vi "read single line.vi"(8 "error in (no error)":errorcluster, 11 "USB IO in":refnum<class "USB IO.lvclass">) -> (0 "error out":errorcluster, 2 "data":bool, 3 "USB IO out":refnum<class "USB IO.lvclass">)   [LabVIEW 2025, in "USB IO.lvclass"]
uses:
  USB IO.lvclass
  USB IO.lvclass/USB IO.ctl
  <vilib>/DAQmx/read.llb/DAQmx Read (Digital Bool 1Line 1Point).vi
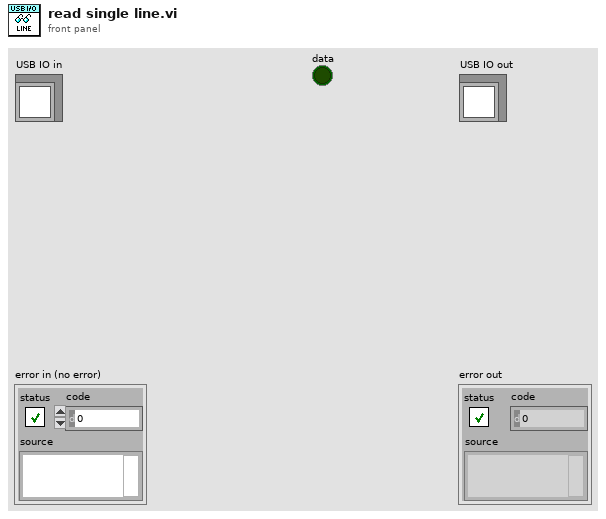
[diagram p1: front panel]
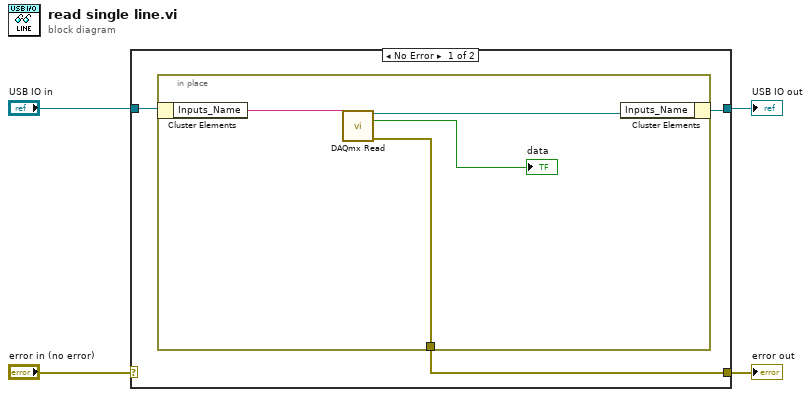
[diagram p0: block diagram]
diagram:
  n1 = case shown="No Error" "error in (no error)" {
    selector: "error in (no error)" -> [_ w13]
    tunnel: [w6 w13] -> w3
    tunnel: [w5 w12] -> w1
    tunnel: "USB IO in" -> [w7 w12]
    frame No Error {
      n2 = in-place {
        in-place-border: [w9] -> w6
        n3 = in-place-cluster #1(w7) -> ("Inputs_Name"=w11:string)
        n4 = call-poly <vilib>:"DAQmx Read.vi"("task/channels in"=w11) -> ("task out"=w10:refnum<k21>, "data"=→"data":bool, "error out"=w9:errorcluster)  [unwired: 12 in]
        n5 = in-place-cluster #1("Inputs_Name"=w10) -> (w5:refnum<class "USB IO.lvclass">)
      }
    }
    frame Error {
    }
  }
  "error out" <- w3
  "USB IO out" <- w1
